vi "Login.vi"() -> ()   [LabVIEW 2023]
uses:
  <vilib>/addons/database/Connection.llb/DB Tools Open Connec (String).vi
  <vilib>/addons/database/Connection.llb/Conn Execute.vi
  <vilib>/addons/database/Recordset.llb/Rec Fetch Recordset Data (R).vi
  <vilib>/addons/database/Recordset.llb/Rec Destroy - Connection.vi
  <vilib>/addons/database/_DB Variant To Data/Database Variant To Data.xnode
  <vilib>/addons/database/NI_Database_API.lvlib
panel:
  out "指示灯":bool
  out "data":string[][](array[string])
  in  "取消":bool
  in  "登录":bool
  in  "密   码：":string
  in  "用户名：":string
  # "登录界面"
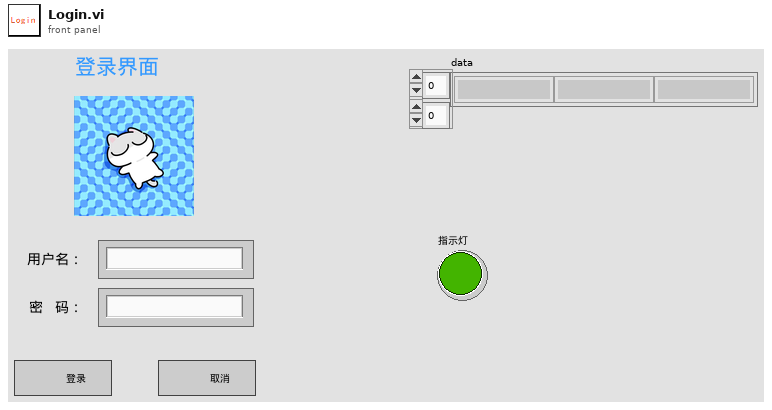
[diagram p1: front panel]
types:
  T1 = typedef "Global Parameter.ctl" = cluster{"User Information":cluster{"用户名：":string, "密   码：":string}, "Login？":bool}
  T2 = typedef "NI_Database_API.lvlib/Conn ObjectReference.ctl" = refnum<k1>
  T3 = typedef "NI_Database_API.lvlib/Rec ObjectReference.ctl" = refnum<k1>
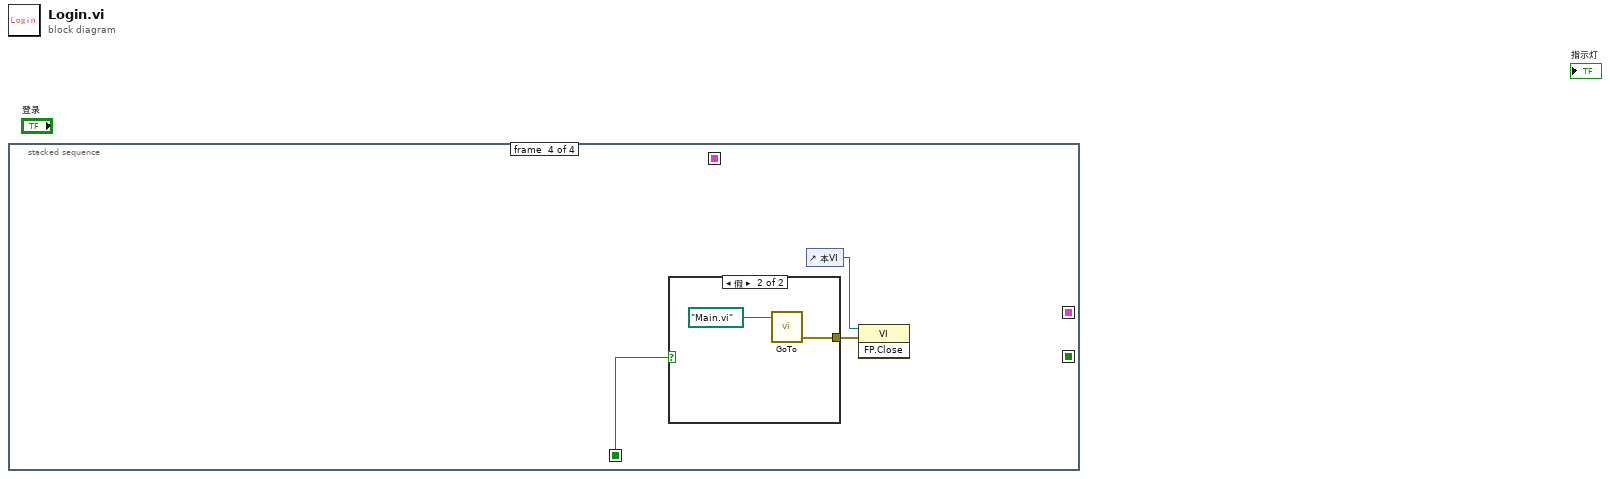
[diagram p0: block diagram]
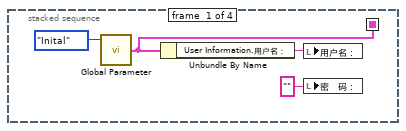
[diagram p2: hidden frame]
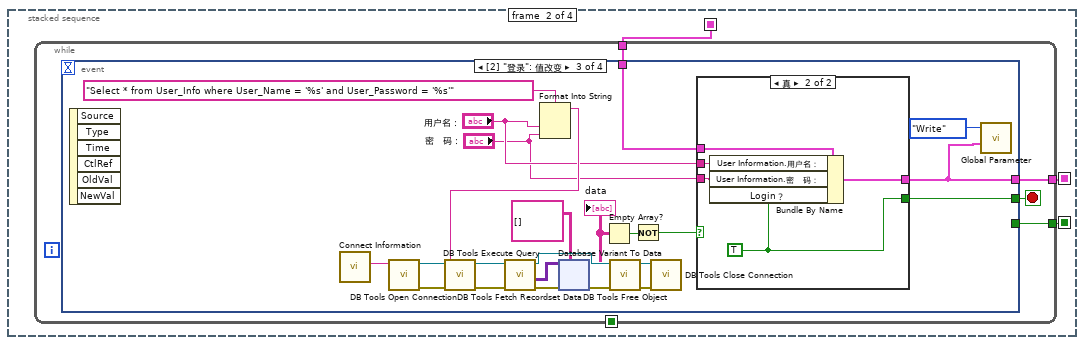
[diagram p3: hidden frame]
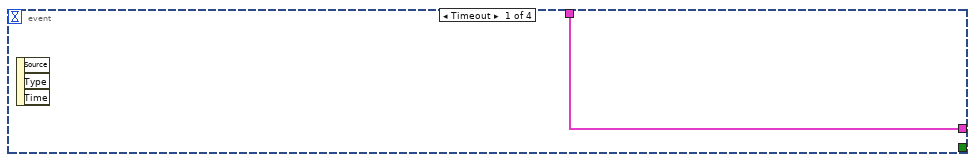
[diagram p4: hidden frame]
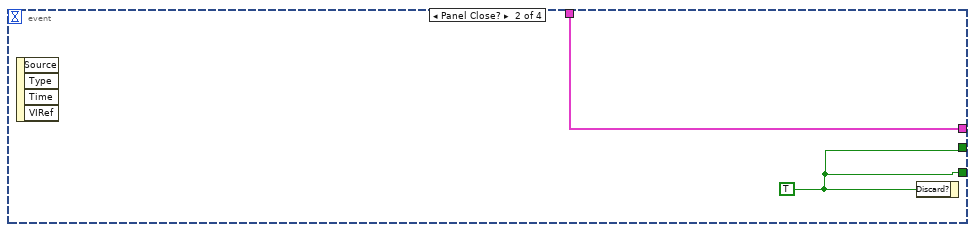
[diagram p5: hidden frame]
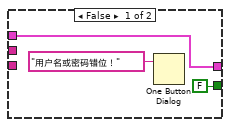
[diagram p6: hidden frame]
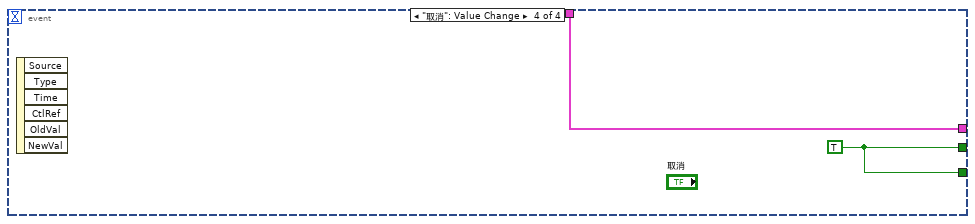
[diagram p7: hidden frame]
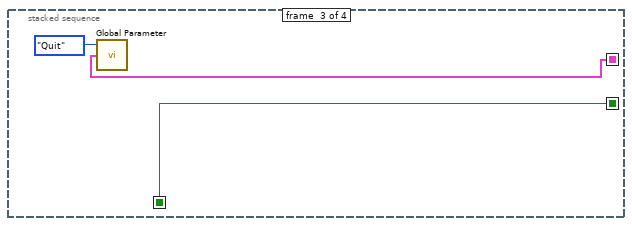
[diagram p8: hidden frame]
diagram:
  n1 = stacked-sequence {
    seq-local: [w1 _ _ _] -> [_ w7 _ _]
    seq-local: [_ w6 _ _] -> [_ _ w93 _]
    seq-local: [_ w5 _ _] -> [_ _ w92 _]
    seq-local: [_ _ w92 _] -> [_ _ _ w97]
    frame #0 {
      n2 = call "Global Parameter.vi"("枚举"=enum16{"Inital", "Read", "Write", "Quit"}."Inital") -> ("Read"=w1:T1)  [unwired: 3 in, 1 out]
      n3 = Unbundle By Name(w1) -> ("User Information.用户名："=w3:string)
      n4 = local write "用户名："(w3) -> ()
      n5 = local write "密   码："("" ("密   码：")) -> ()
    }
    frame #1 {
      n6 = while {
        tunnel: w7 -> [w10]
        tunnel: [w9] -> w6
        tunnel: [w8] -> w5
        stop <- w11 stop-if-true
        n7 = event shown="[2] \"登录\": 值改变" {
          selector: _ -> [_ _ _ _]
          dyn-events: _ -> [_ _ _ _]
          timeout: _ -> [_ _ _ _]
          tunnel: [_ w13 w20 w90] -> w11
          tunnel: w10 -> [w12 w14 w19 w91]
          tunnel: [w12 w14 w15 w91] -> w9
          tunnel: [_ w13 _ w90] -> w8
          event Timeout {
            n8 = event-data() -> ()  [unwired: 1 in, 3 out]
          }
          event Panel Close? {
            w13 = TRUE
            n9 = event-data() -> ()  [unwired: 1 in, 4 out]
            n10 = event-data("Discard?"=w13) -> ()  [unwired: 1 in, 1 out]
          }
          event "登录": Value Change {
            n11 = event-data() -> ()  [unwired: 1 in, 6 out]
            n12 = call "Connect Information.vi"() -> ("Connect Info"=w37:string)  [unwired: 11 in]
            n13 = call-poly <vilib>:"DB Tools Open Connection.vi"("connection information"=w37) -> ("error out"=w29:errorcluster, "connection reference"=w30:T2)  [unwired: 7 in]
            n14 = Format Into String(format string="Select * from User_Info where User_Name = '%s' and User_Password = '%s'" ("SQL query"), "用户名：", "密   码：") -> (resulting string=w25:string)  [unwired: 2 in, 1 out]
            n15 = call-poly <vilib>:"DB Tools Execute Query.vi"("error in (no error)"=w29, "SQL query"=w25, "connection reference"=w30) -> ("error out"=w27:errorcluster, "recordset reference"=w28:T3)  [unwired: 5 in]
            n16 = call-poly <vilib>:"DB Tools Fetch Recordset Data.vi"("error in (no error)"=w27, "recordset reference"=w28) -> ("error out"=w31:errorcluster, "recordset data"=w32:variant[][], "recordset reference out"=w35:T3)  [unwired: 3 in]
            n17 = xnode "Database Variant To Data"("database variant"=w32, "error in (no error)"=w31, "type"=string[][] []) -> ("data"=w23:string[][], "error out"=w33:errorcluster)
            "data" <- w23
            n18 = Empty Array?(array=w23) -> (empty?=w22:bool)
            n19 = call-poly <vilib>:"DB Tools Free Object.vi"("error in (no error)"=w33, "recordset reference"=w35) -> ("error out"=w34:errorcluster, "connection reference"=w36:T2)  [unwired: 8 in]
            n20 = Not(x=w22) -> (.not. x?=w21:bool)
            n21 = call <vilib>:"DB Tools Close Connection.vi"("error in (no error)"=w34, "connection reference"=w36) -> ()  [unwired: 5 in, 1 out]
            n22 = case shown="真" w21 {
              tunnel: [FALSE w41] -> w20
              tunnel: w19 -> [w39 w45]
              tunnel: "用户名：" -> [_ w44]
              tunnel: "密   码：" -> [_ w43]
              tunnel: [w39 w42] -> w15
              frame False {
                n23 = One Button Dialog(message="用户名或密码错位！" ("消息")) -> ()  [unwired: 1 in, 1 out]
              }
              frame True {
                w41 = TRUE
                n24 = Bundle By Name(cluster=w45, "User Information.用户名："=w44, "User Information.密   码："=w43, "Login？"=w41) -> (w42:T1)
              }
            }
            n25 = call "Global Parameter.vi"("Write"=w15, "枚举"=enum16{"Inital", "Read", "Write", "Quit"}."Write") -> ()  [unwired: 2 in, 2 out]
          }
          event "取消": Value Change {
            w90 = TRUE
            n26 = event-data() -> ()  [unwired: 1 in, 6 out]
          }
        }
      }
    }
    frame #2 {
      n27 = call "Global Parameter.vi"("Write"=w93, "枚举"=enum16{"Inital", "Read", "Write", "Quit"}."Quit") -> ()  [unwired: 2 in, 2 out]
    }
    frame #3 {
      n28 = case shown="假" w97 {
        tunnel: [_ w98] -> w95
        frame True {
        }
        frame False {
          n29 = call "GoTo.vi"("名称或相对路径"=path "Main.vi") -> ("错误输出"=w98:errorcluster)  [unwired: 4 in]
        }
      }
      n30 = control-ref of="本VI"() -> (w96:refnum<vi>)
      n31 = invoke class="VI" method="FP.Close"(reference=w96, error in=w95) -> ()  [unwired: 1 in, 3 out]
    }
  }
